vi "Simulation-Drehstrom.vi"() -> ()   [LabVIEW 2015]
uses:
  <vilib>/Math Plots/2D Math Plots/2D Compass/2D Compass XCtrl/2D Compass.xctl
  <vilib>/measure/matone.llb/Extract Single Tone Information 1 Chan.vi
  <vilib>/Math Plots/2D Math Plots/2D Compass/2D Compass Datatype/Public/Plot Helper (Vector).vi
  <vilib>/measure/NI_MABase.lvlib
  <vilib>/measure/NI_MAPro.lvlib
  <vilib>/Math Plots/2D Math Plots/2D Compass/2D Compass Datatype/2D Compass Datatype.lvclass
panel:
  out "Angehängtes Array":dbl[][](array[numeric])
  out "Frequenz 3":dbl
  out "Frequenz 2":dbl
  out "Phase 3":dbl
  out "Amplitude 3":dbl
  out "Phase 2":dbl
  out "Amplitude 2":dbl
  out "Phase 1":dbl
  out "Amplitude 1":dbl
  out "Frequenz 1":dbl
  in  "Phase 1":dbl
  in  "Frequenz 3":dbl=50.0
  in  "Frequenz 2":dbl=50.0
  in  "Frequenz 1":dbl=50.0
  in  "Amplitude 3":dbl=230.0
  in  "Amplitude 2":dbl=230.0
  in  "Amplitude 1":dbl=230.0
  out "2D Compass":refnum<class "2D Plot Datatype.lvclass">[](xcontrol) caption="2D-Kompass"
  in  "Phase 3":dbl=240.0
  in  "Phase 2":dbl=120.0
  # "Parameter Eingabepanel"
  # "Messwerte Ausgabewerte"
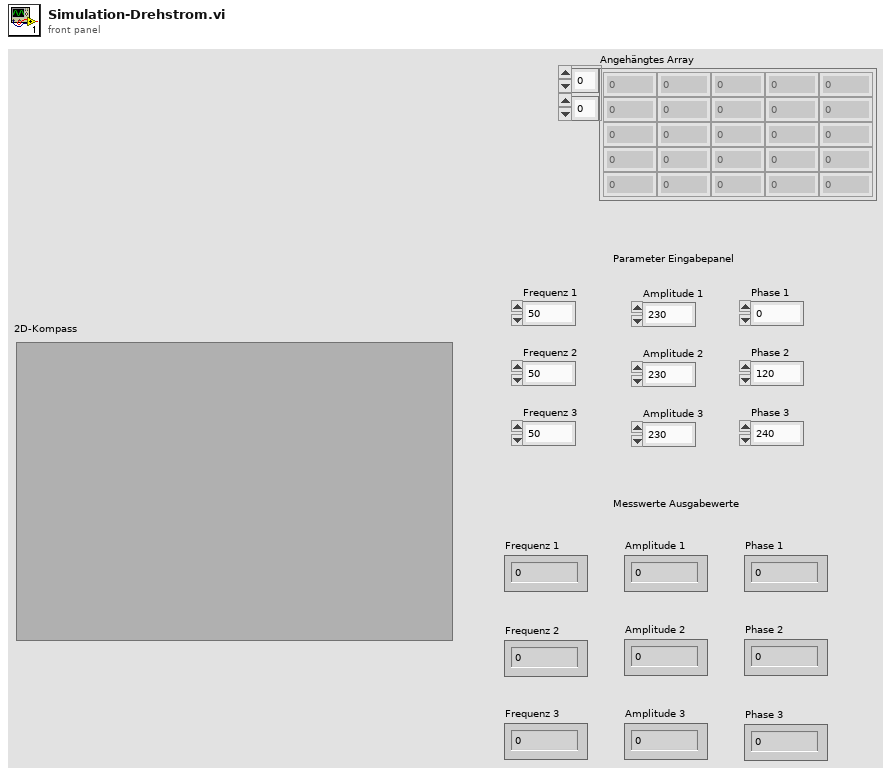
[diagram p1: front panel]
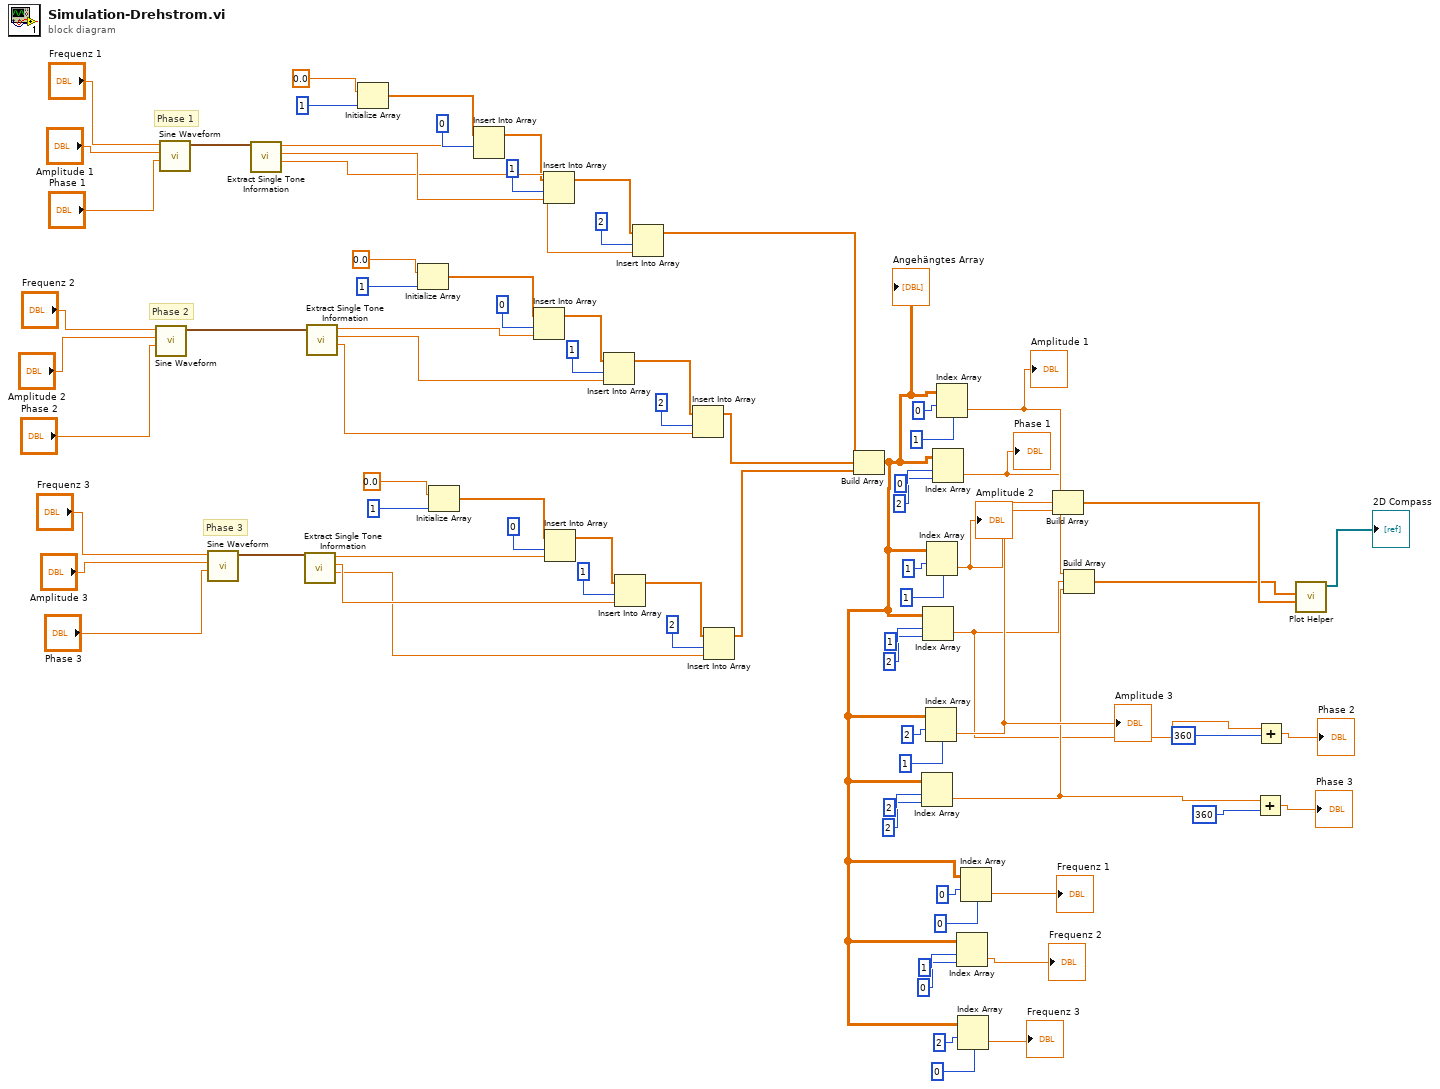
[diagram p0: block diagram]
diagram:
  # "Phase 3"
  # "Phase 2"
  # "Phase 1"
  n1 = call <vilib>:"Sine Waveform.vi"("phase"="Phase 2", "amplitude"="Amplitude 2", "frequency"="Frequenz 2") -> ("signal out"=w82:waveform(dbl))  [unwired: 7 in, 1 out]
  n2 = call <vilib>:"Sine Waveform.vi"("phase"="Phase 1", "amplitude"="Amplitude 1", "frequency"="Frequenz 1") -> ("signal out"=w81:waveform(dbl))  [unwired: 7 in, 1 out]
  n3 = call <vilib>:"Sine Waveform.vi"("phase"="Phase 3", "amplitude"="Amplitude 3", "frequency"="Frequenz 3") -> ("signal out"=w72:waveform(dbl))  [unwired: 7 in, 1 out]
  n4 = call-poly <vilib>:"Extract Single Tone Information.vi"("time signal in"=w81) -> ("detected phase (deg)"=w66:dbl, "detected amplitude"=w67:dbl, "detected frequency"=w70:dbl)  [unwired: 5 in, 3 out]
  n5 = call-poly <vilib>:"Extract Single Tone Information.vi"("time signal in"=w72) -> ("detected phase (deg)"=w39:dbl, "detected amplitude"=w40:dbl, "detected frequency"=w41:dbl)  [unwired: 5 in, 3 out]
  n6 = call-poly <vilib>:"Extract Single Tone Information.vi"("time signal in"=w82) -> ("detected phase (deg)"=w50:dbl, "detected amplitude"=w51:dbl, "detected frequency"=w52:dbl)  [unwired: 5 in, 3 out]
  n7 = Initialize Array(0.0, 1) -> (w64:dbl[])
  n8 = Initialize Array(0.0, 1) -> (w56:dbl[])
  n9 = Initialize Array(0.0, 1) -> (w45:dbl[])
  n10 = Insert Into Array(array=w64, index=0, new element=w70) -> (w62:dbl[])
  n11 = Insert Into Array(array=w56, index=0, new element=w52) -> (w54:dbl[])
  n12 = Insert Into Array(array=w62, index=1, new element=w67) -> (w61:dbl[])
  n13 = Insert Into Array(array=w45, index=0, new element=w41) -> (w43:dbl[])
  n14 = Insert Into Array(array=w54, index=1, new element=w51) -> (w53:dbl[])
  n15 = Insert Into Array(array=w43, index=1, new element=w40) -> (w42:dbl[])
  n16 = Insert Into Array(array=w61, index=2, new element=w66) -> (w38:dbl[])
  n17 = Insert Into Array(array=w53, index=2, new element=w50) -> (w37:dbl[])
  n18 = Insert Into Array(array=w42, index=2, new element=w39) -> (w36:dbl[])
  n19 = Build Array(w38, w37, w36) -> (w10:dbl[][])
  "Angehängtes Array" <- w10
  n20 = Index Array(array=w10, index (row)=2, index (col)=2) -> (element=w4:dbl)
  n21 = Index Array(array=w10, index (row)=1, index (col)=2) -> (element=w3:dbl)
  n22 = Index Array(array=w10, index (row)=2, index (col)=1) -> (element=w17:dbl)
  "Amplitude 3" <- w17
  n23 = Index Array(array=w10, index (row)=1, index (col)=1) -> (element=w18:dbl)
  "Amplitude 2" <- w18
  n24 = Index Array(array=w10, index (row)=0, index (col)=2) -> (element=w19:dbl)
  "Phase 1" <- w19
  n25 = Index Array(array=w10, index (row)=0, index (col)=1) -> (element=w20:dbl)
  "Amplitude 1" <- w20
  n26 = Index Array(array=w10, index (row)=1, index (col)=0) -> (element=→"Frequenz 2":dbl)
  n27 = Index Array(array=w10, index (row)=2, index (col)=0) -> (element=→"Frequenz 3":dbl)
  n28 = Index Array(array=w10, index (row)=0, index (col)=0) -> (element=→"Frequenz 1":dbl)
  n29 = Build Array(w20, w18, w17) -> (w23:dbl[])
  n30 = Build Array(w19, w3, w4) -> (w22:dbl[])
  n31 = Add(x=w4, y=360) -> (x+y=→"Phase 3":dbl)
  n32 = Add(x=w3, y=360) -> (x+y=→"Phase 2":dbl)
  n33 = call-poly <vilib>:"Plot Helper.vi"("radius vector"=w23, "theta vector"=w22) -> ("2D Plot Class Obj Array out"=→"2D Compass":refnum<class "2D Plot Datatype.lvclass">[])  [unwired: 2 in, 7 out]
